vi "UserView_Entry_Console.vi"(8 "error in":errorcluster) -> (0 "error out":errorcluster)   [LabVIEW 2019]
uses:
  #typedef_Queue_enum.ctl
  #typedef_EntryConsole_Action_enum.ctl
  #typedef_Data_Controller.ctl
  #typedef_WashDisplay_Action_enum.ctl
  #typedef_Controller_Action_enum.ctl
  #typedef_VehiclePosition_Action_enum.ctl
  #typedef_VehiclePos_enum.ctl
  #typedef_WashStepInfo.ctl
  #typedef_WashStates.ctl
  #typedef_Data_Entry.ctl
panel:
  in  "Start":bool
  in  "Air Dry":bool
  in  "Tire Shine Foam":bool
  in  "Spot Free Rinse":bool
  in  "Low Pressure Wax":bool
  in  "High Pressure Wash (default)":bool
  in  "Pre-Soak":bool
  in  "Bug Remover":bool
  in  "Under Body Wash":bool
  # "Entry Console"
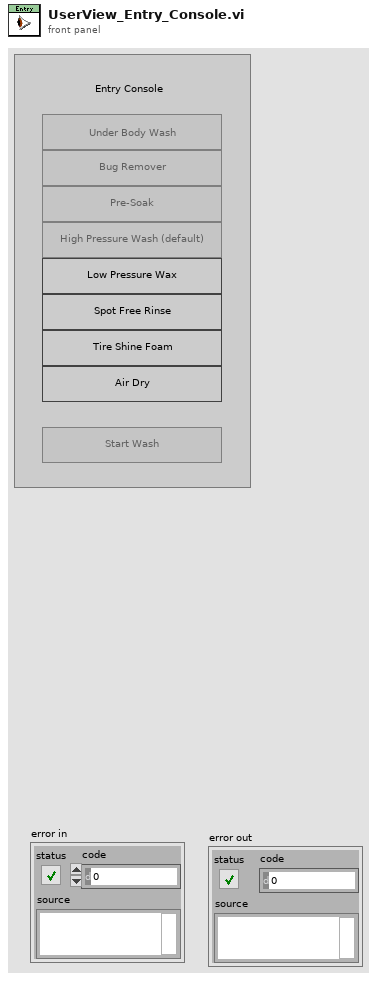
[diagram p1: front panel]
types:
  T1 = typedef "#typedef_Queue_enum.ctl" = enum16{"ERROR_default", "Obtain", "Enqueue", "GetStatus", "Flush", "Release"}
  T2 = typedef "#typedef_Data_Entry.ctl" = cluster{"Under Body Wash":bool, "Bug Remover":bool, "Pre-Soak":bool, "High Pressure Wash (default)":bool, "Low Pressure Wax":bool, "Spot Free Rinse":bool, "Tire Shine Foam":bool, "Air Dry":bool, "Start":bool, "EntryConsole_Action":T3}
  T3 = typedef "#typedef_EntryConsole_Action_enum.ctl" = enum16{"Init", "ERROR_DEFAULT", "Idle", "Start_Wash_Cycle", "Clear_Console", "Close", "Error_Handler", "Exit"}
  T4 = typedef "#typedef_Data_Controller.ctl" = cluster{"EntryConsole_Action":T3, "WashDisplay_Action":T5, "Controller_Action":T6, "VehiclePosition_Action":T7, "Under Body Wash":bool, "Bug Remover":bool, "Pre-Soak":bool, "High Pressure Wash (default)":bool, "Low Pressure Wax":bool, "Spot Free Rinse":bool, "Tire Shine Foam":bool, "Air Dry":bool, "Start":bool, "Current Vehicle Pos":T8, "Steps List":T9[], "Current Step Ind":i32}
  T5 = typedef "#typedef_WashDisplay_Action_enum.ctl" = enum16{"Init", "ERROR_DEFAULT", "Idle", "Update FP", "Close", "Error_Handler", "Exit"}
  T6 = typedef "#typedef_Controller_Action_enum.ctl" = enum16{"ERROR_DEFAULT", "Init", "Read database", "(Idle) Wait for Start", "Start", "Wait for Vehicle Pos", "Wash Step Execution", "Wash Completion", "Wash Exit", "Wash Abort", "Close", "Error Handler", "Exit"}
  T7 = typedef "#typedef_VehiclePosition_Action_enum.ctl" = enum16{"Init", "ERROR_DEFAULT", "Idle", "Close", "Error_Handler", "Exit", "Send Vehicle Pos"}
  T8 = typedef "#typedef_VehiclePos_enum.ctl" = u8
  T9 = typedef "#typedef_WashStepInfo.ctl" = cluster{"Wash States":T10, "Expected Vehicle Pos":i32, "Step duration":i32}
  T10 = typedef "#typedef_WashStates.ctl" = enum16{"Under Body Wash", "Bug Remover", "Pre-Soak", "High Pressure Wash", "Low Pressure Wax", "Spot Free Rinse", "Tire Shine Foam", "Air Dry"}
  T11 = enum8{"Enabled", "Disabled", "Disabled and Grayed Out"}
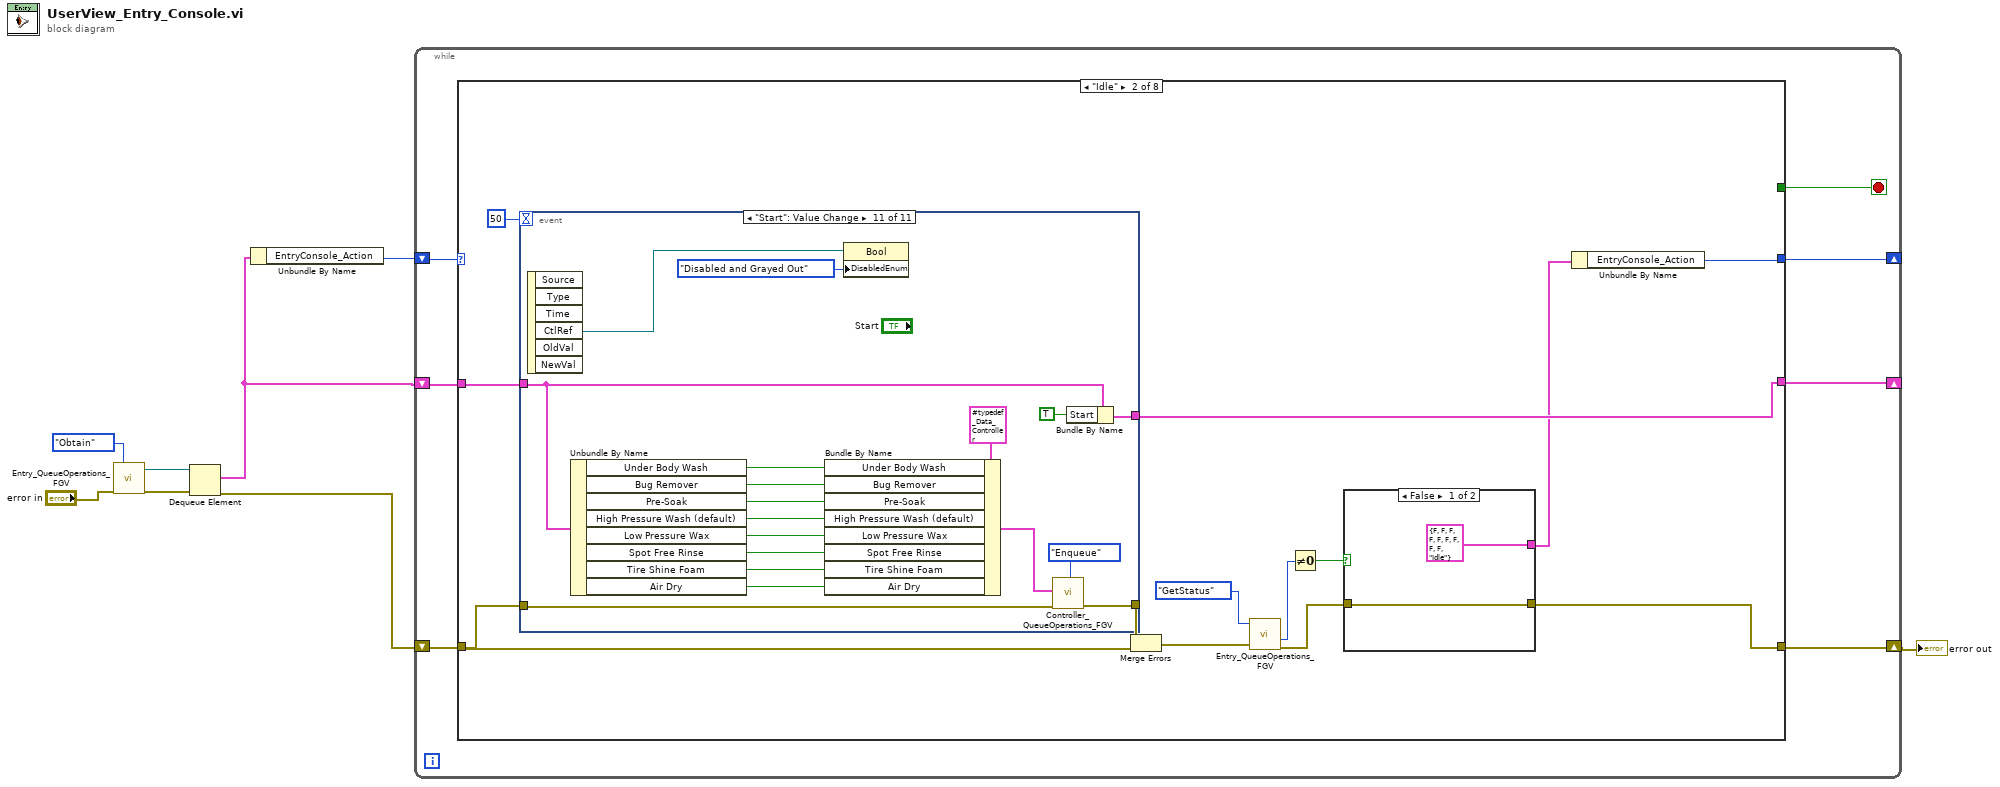
[diagram p0: block diagram]
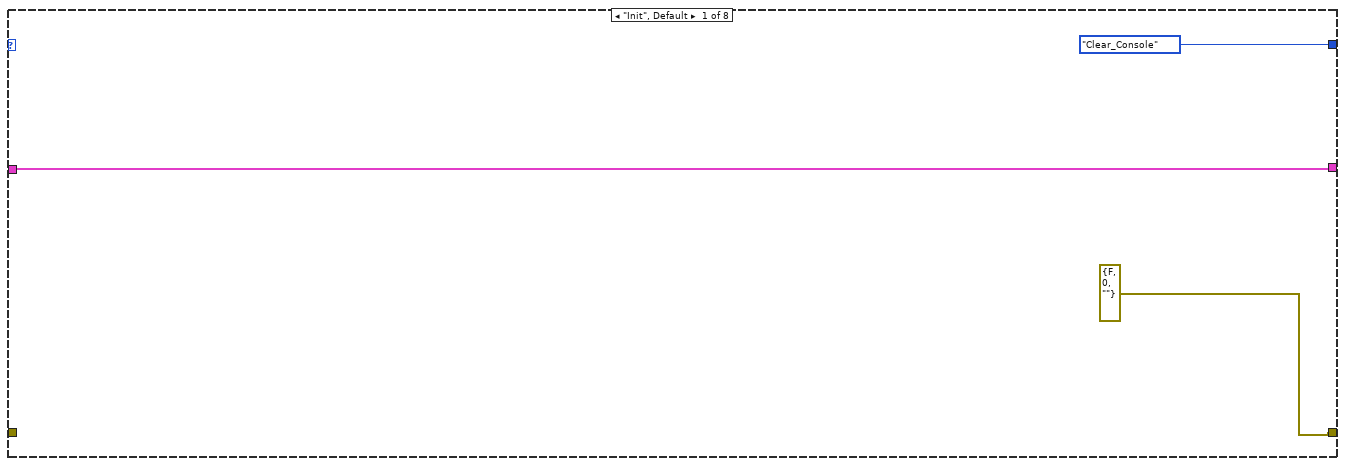
[diagram p2: hidden frame]
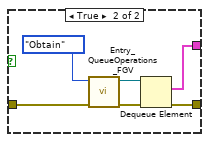
[diagram p3: hidden frame]
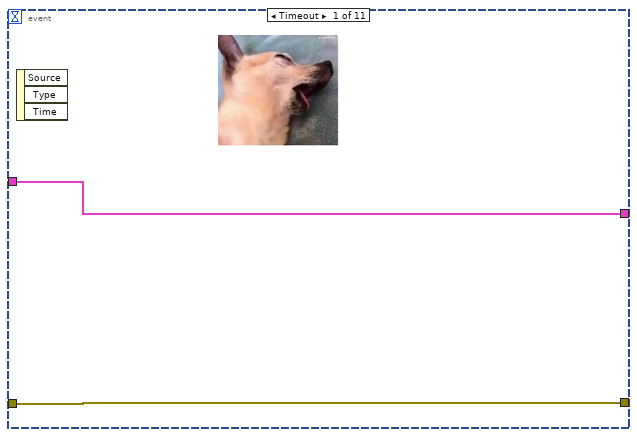
[diagram p4: hidden frame]
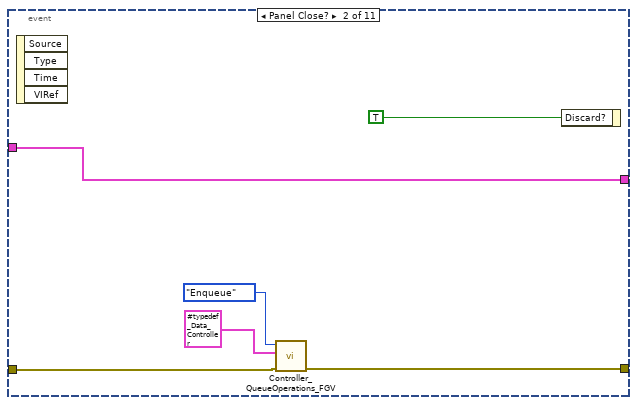
[diagram p5: hidden frame]
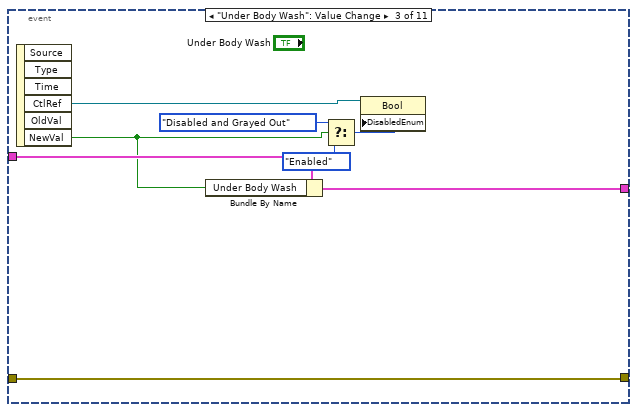
[diagram p6: hidden frame]
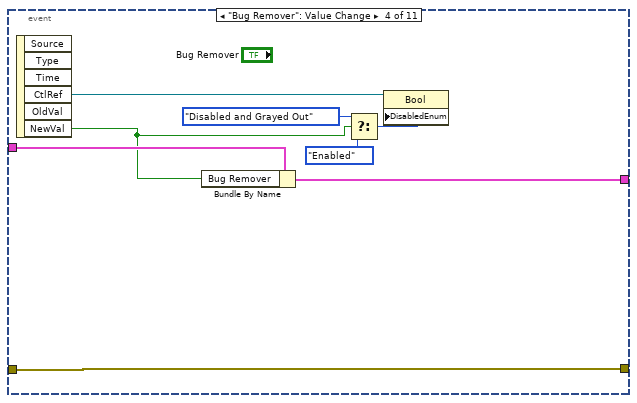
[diagram p7: hidden frame]
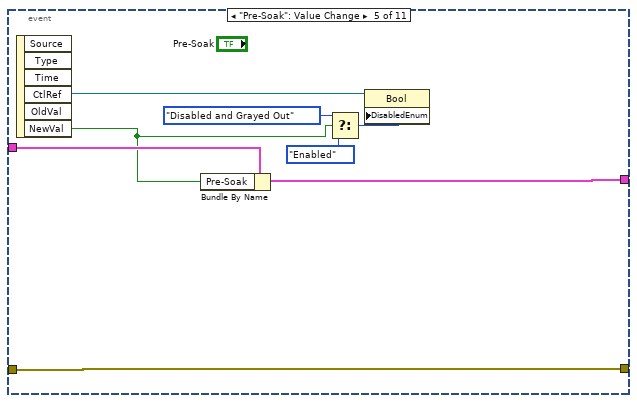
[diagram p8: hidden frame]
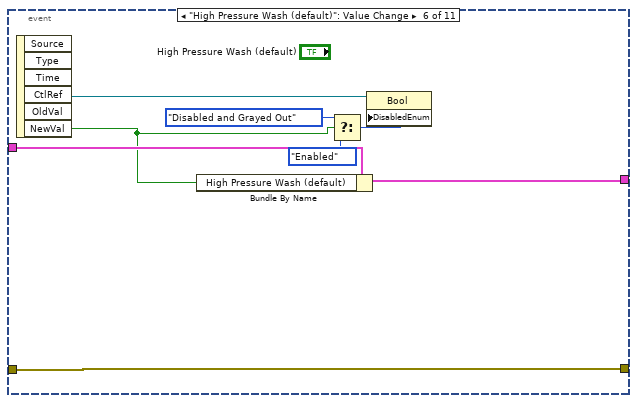
[diagram p9: hidden frame]
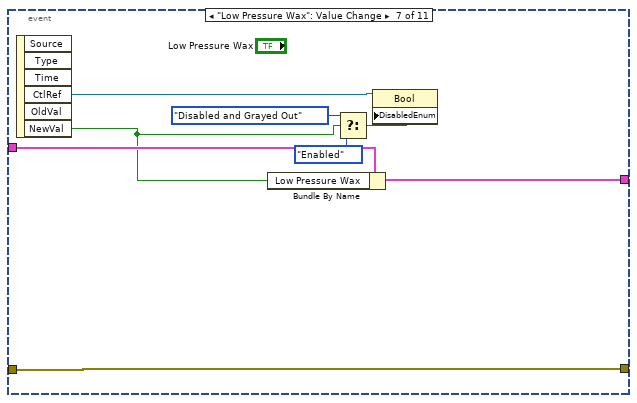
[diagram p10: hidden frame]
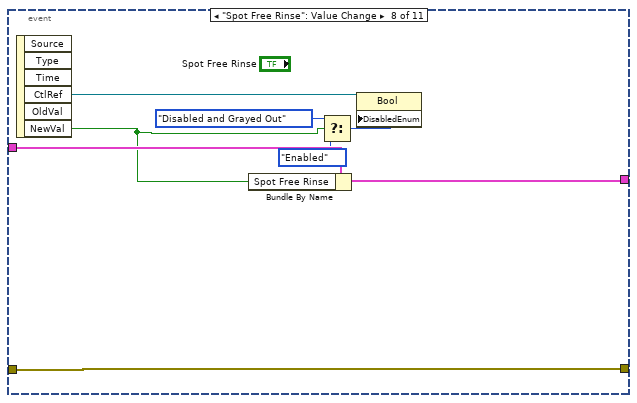
[diagram p11: hidden frame]
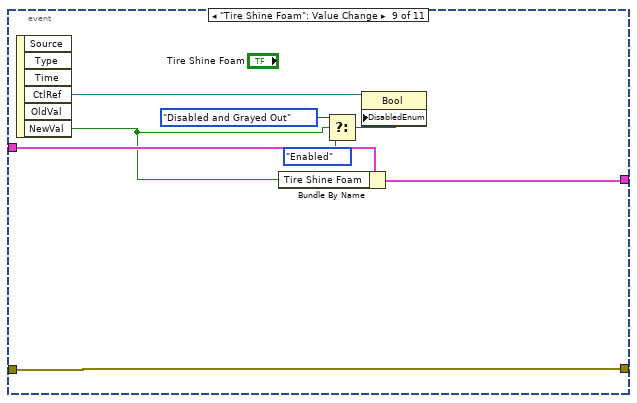
[diagram p12: hidden frame]
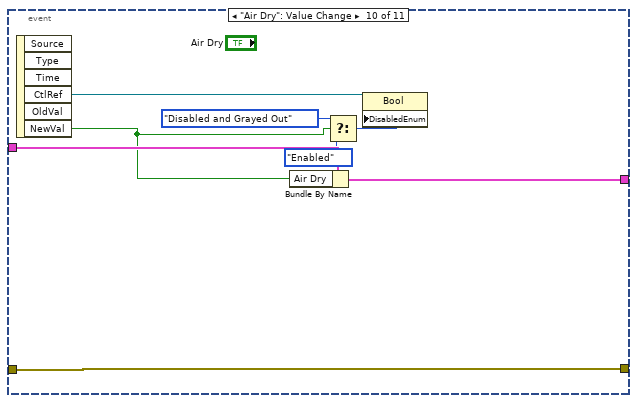
[diagram p13: hidden frame]
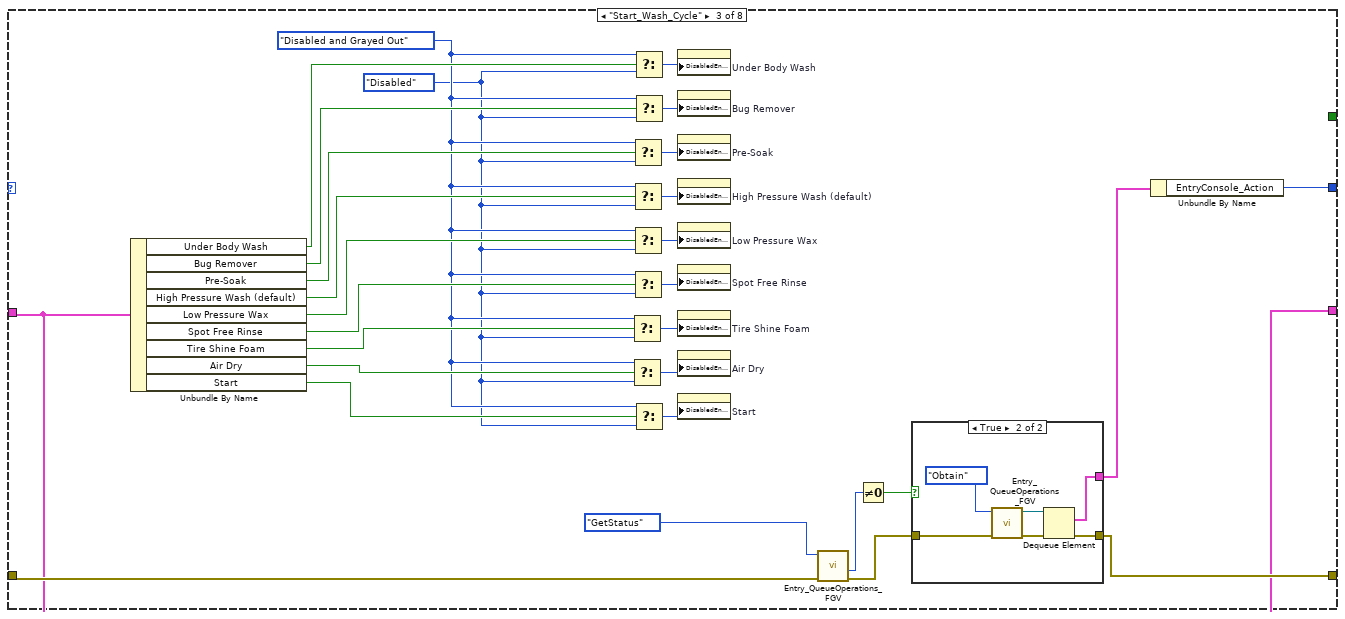
[diagram p14: hidden frame]
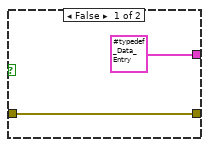
[diagram p15: hidden frame]
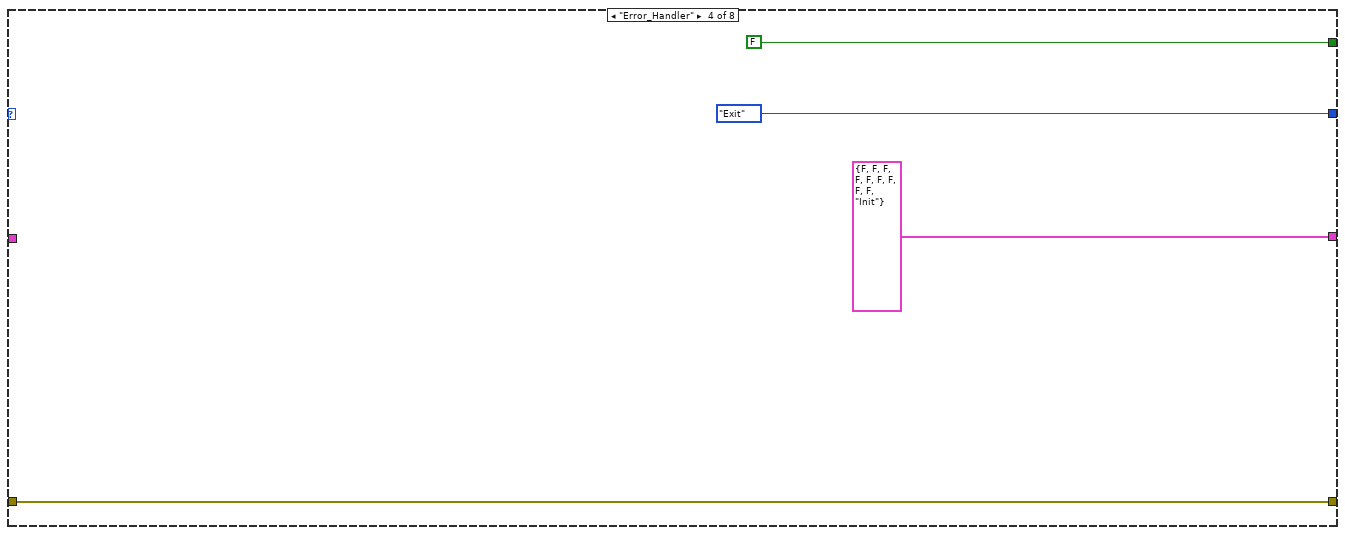
[diagram p16: hidden frame]
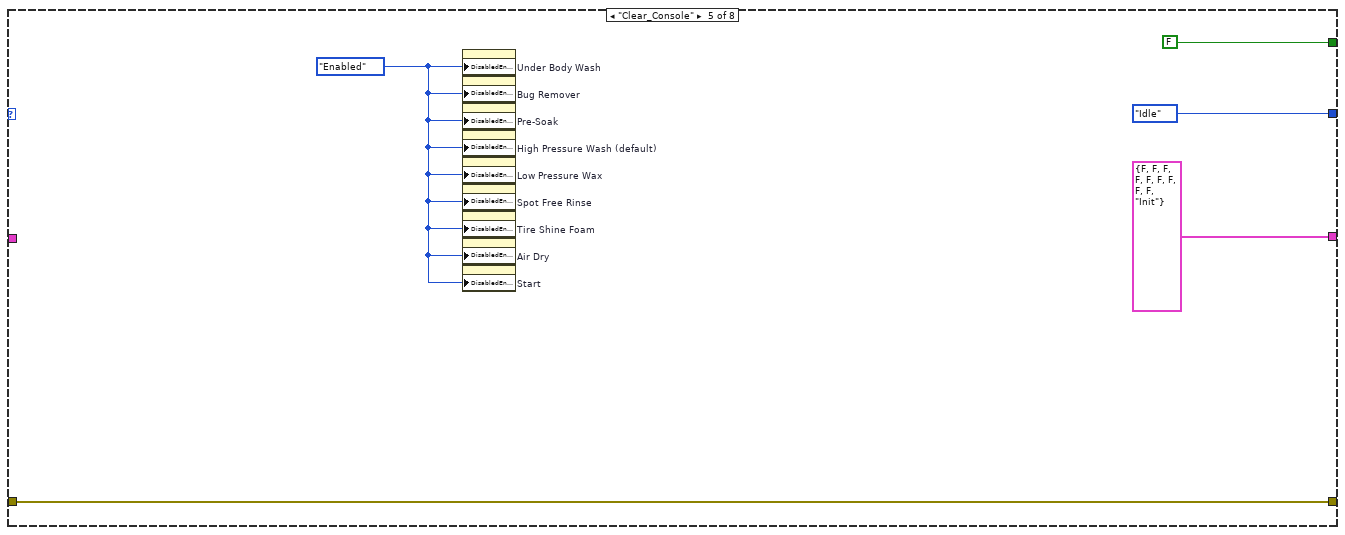
[diagram p17: hidden frame]
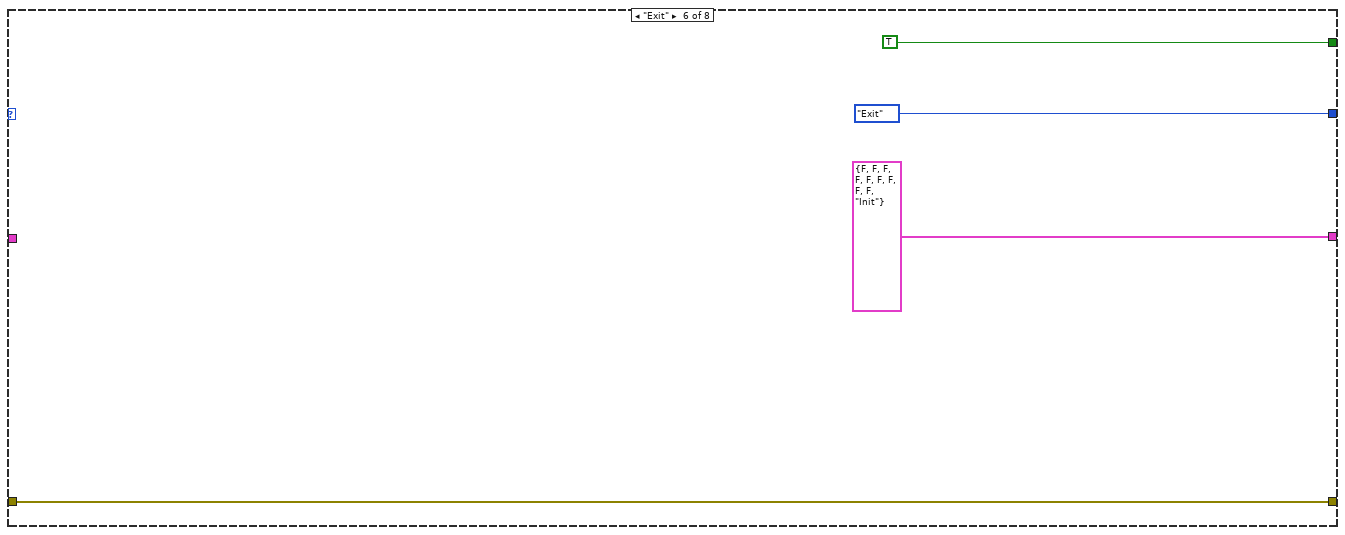
[diagram p18: hidden frame]
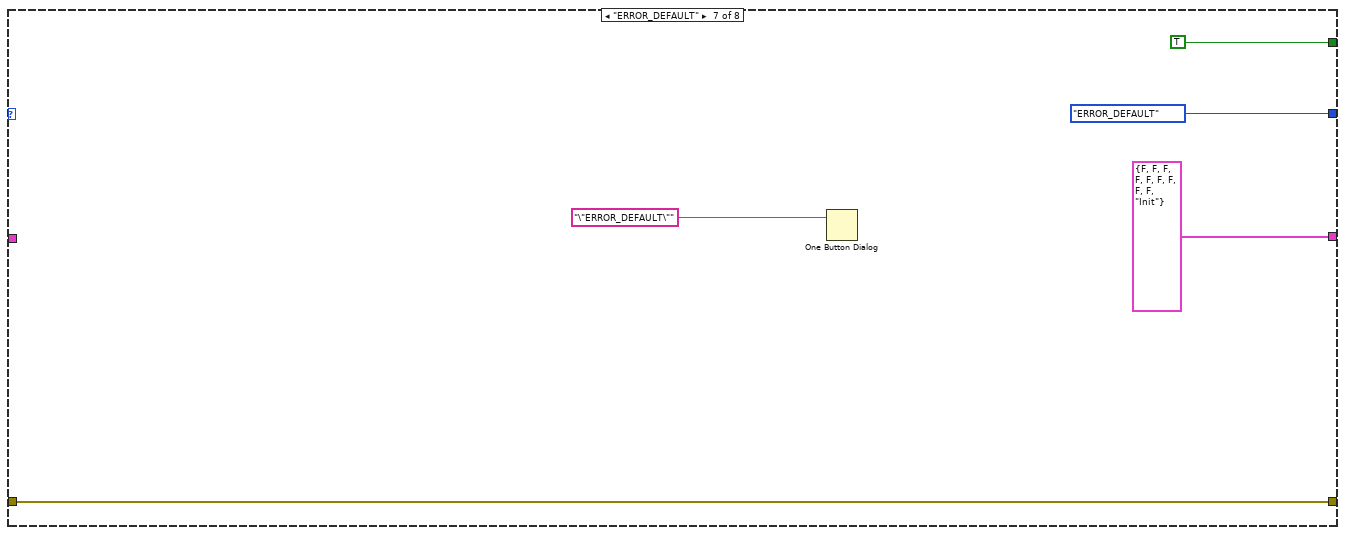
[diagram p19: hidden frame]
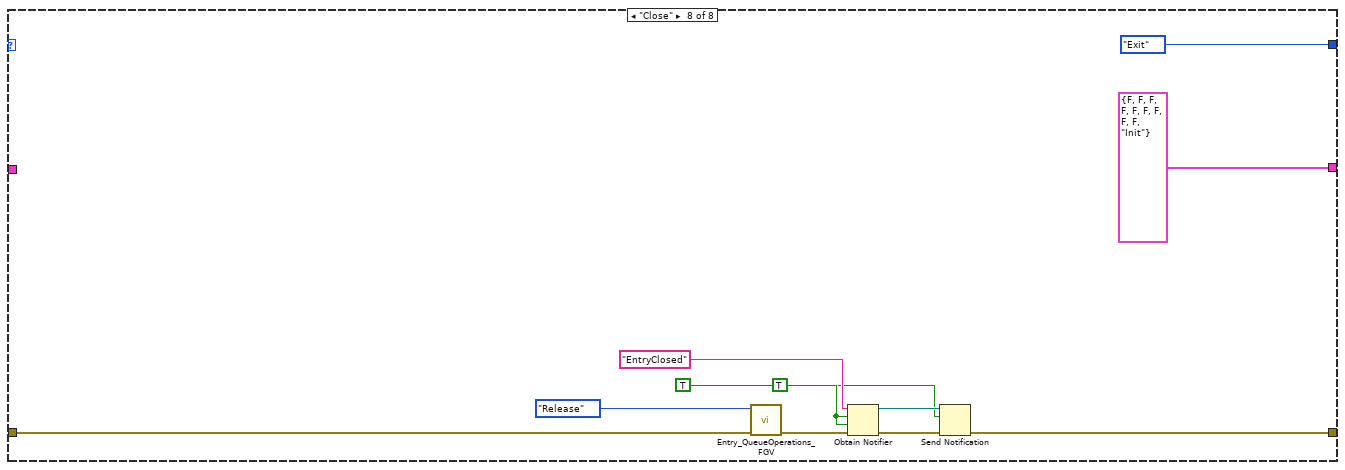
[diagram p20: hidden frame]
diagram:
  n1 = call "Entry_QueueOperations_FGV.vi"("error in"="error in", "Action"=#typedef_Queue_enum."Obtain") -> ("error out"=w5:errorcluster, "queue ref"=w6:refnum<queue>)  [unwired: 6 in, 2 out]
  n2 = Dequeue Element(queue=w6, error in (no error)=w5) -> (element=w4:T2, error out=w2:errorcluster)  [unwired: 1 in, 2 out]
  n3 = Unbundle By Name(w4) -> ("EntryConsole_Action"=w3:T3)
  n4 = while {
    shift-right: [w14] -> _
    shift-left: w3 -> [w15]
    shift-right: [w12] -> _
    shift-left: w4 -> [w9]
    shift-right: [w10] -> w1
    shift-left: w2 -> [w11]
    stop <- w13 stop-if-true
    n5 = case shown="\"Idle\"" w15 {
      tunnel: [#typedef_EntryConsole_Action_enum."Clear_Console" w25 w131 #typedef_EntryConsole_Action_enum."Exit" #typedef_EntryConsole_Action_enum."Idle" #typedef_EntryConsole_Action_enum."Exit" #typedef_EntryConsole_Action_enum."ERROR_DEFAULT" #typedef_EntryConsole_Action_enum."Exit"] -> w14
      tunnel: [_ _ _ FALSE FALSE TRUE TRUE _] -> w13
      tunnel: [w16 w26 w130 T2 {"Under Body Wash"=FALSE, "Bug Remover"=FALSE, "Pre-Soak"=FALSE, "High Pressure Wash (default)"=FALSE, "Low Pressure Wax"=FALSE, "Spot Free Rinse"=FALSE, "Tire Shine Foam"=FALSE, "Air Dry"=FALSE, "Start"=FALSE, "EntryConsole_Action"=enum."Init"} ("Data") T2 {"Under Body Wash"=FALSE, "Bug Remover"=FALSE, "Pre-Soak"=FALSE, "High Pressure Wash (default)"=FALSE, "Low Pressure Wax"=FALSE, "Spot Free Rinse"=FALSE, "Tire Shine Foam"=FALSE, "Air Dry"=FALSE, "Start"=FALSE, "EntryConsole_Action"=enum."Init"} ("Data") T2 {"Under Body Wash"=FALSE, "Bug Remover"=FALSE, "Pre-Soak"=FALSE, "High Pressure Wash (default)"=FALSE, "Low Pressure Wax"=FALSE, "Spot Free Rinse"=FALSE, "Tire Shine Foam"=FALSE, "Air Dry"=FALSE, "Start"=FALSE, "EntryConsole_Action"=enum."Init"} ("Data") T2 {"Under Body Wash"=FALSE, "Bug Remover"=FALSE, "Pre-Soak"=FALSE, "High Pressure Wash (default)"=FALSE, "Low Pressure Wax"=FALSE, "Spot Free Rinse"=FALSE, "Tire Shine Foam"=FALSE, "Air Dry"=FALSE, "Start"=FALSE, "EntryConsole_Action"=enum."Init"} ("Data") T2 {"Under Body Wash"=FALSE, "Bug Remover"=FALSE, "Pre-Soak"=FALSE, "High Pressure Wash (default)"=FALSE, "Low Pressure Wax"=FALSE, "Spot Free Rinse"=FALSE, "Tire Shine Foam"=FALSE, "Air Dry"=FALSE, "Start"=FALSE, "EntryConsole_Action"=enum."Init"} ("Data")] -> w12
      tunnel: w11 -> [_ w28 w132 w168 w173 w178 w181 w192]
      tunnel: [errorcluster {"status"=FALSE, "code"=0, "source"=""} ("error constant") w21 w133 w168 w173 w178 w181 w188] -> w10
      tunnel: w9 -> [w16 w27 w130 _ _ _ _ _]
      frame "Init", Default {
      }
      frame "Idle" {
        n6 = event shown="[10] \"Start\": Value Change" {
          selector: _ -> [_ _ _ _ _ _ _ _ _ _ _]
          dyn-events: _ -> [_ _ _ _ _ _ _ _ _ _ _]
          timeout: 50 -> [_ _ _ _ _ _ _ _ _ _ _]
          tunnel: w28 -> [w41 w45 w55 w63 w71 w79 w87 w95 w103 w111 w112]
          tunnel: [w41 w44 w55 w63 w71 w79 w87 w95 w103 w111 w125] -> w29
          tunnel: w27 -> [w40 w42 w54 w62 w70 w78 w86 w94 w102 w110 w122]
          tunnel: [w40 w42 w53 w61 w69 w77 w85 w93 w101 w109 w123] -> w26
          event Timeout {
            n7 = event-data() -> ()  [unwired: 1 in, 3 out]
          }
          event Panel Close? {
            n8 = event-data() -> ()  [unwired: 1 in, 4 out]
            n9 = call "Controller_QueueOperations_FGV.vi"("error in"=w45, "Data In"=T4 {"EntryConsole_Action"=enum."Init", "WashDisplay_Action"=enum."Init", "Controller_Action"=enum."Close", "VehiclePosition_Action"=enum."Init", "Under Body Wash"=FALSE, "Bug Remover"=FALSE, "Pre-Soak"=FALSE, "High Pressure Wash (default)"=FALSE, "Low Pressure Wax"=FALSE, "Spot Free Rinse"=FALSE, "Tire Shine Foam"=FALSE, "Air Dry"=FALSE, "Start"=FALSE, "Current Vehicle Pos"=1, "Steps List"=[], "Current Step Ind"=0} ("Data"), "Action"=#typedef_Queue_enum."Enqueue") -> ("error out"=w44:errorcluster)  [unwired: 5 in, 3 out]
            n10 = event-data("Discard?"=TRUE) -> ()  [unwired: 1 in, 1 out]
          }
          event "Under Body Wash": Value Change {
            n11 = event-data() -> ("CtlRef"=w49:refnum<vi>, "NewVal"=w48:bool)  [unwired: 1 in, 4 out]
            n12 = Bundle By Name(cluster=w54, "Under Body Wash"=w48) -> (w53:T2)
            n13 = Select(t=T11."Disabled and Grayed Out" ("Disabled"), s=w48, f=T11."Enabled") -> (s? t:f=w51:T11)
            n14 = property class="Bool"(reference=w49, "DisabledEnum"=w51) -> ()  [unwired: 1 in, 2 out]
          }
          event "Bug Remover": Value Change {
            n15 = event-data() -> ("CtlRef"=w60:refnum<vi>, "NewVal"=w56:bool)  [unwired: 1 in, 4 out]
            n16 = Bundle By Name(cluster=w62, "Bug Remover"=w56) -> (w61:T2)
            n17 = Select(t=T11."Disabled and Grayed Out" ("Disabled"), s=w56, f=T11."Enabled") -> (s? t:f=w58:T11)
            n18 = property class="Bool"(reference=w60, "DisabledEnum"=w58) -> ()  [unwired: 1 in, 2 out]
          }
          event "Pre-Soak": Value Change {
            n19 = event-data() -> ("CtlRef"=w65:refnum<vi>, "NewVal"=w64:bool)  [unwired: 1 in, 4 out]
            n20 = Bundle By Name(cluster=w70, "Pre-Soak"=w64) -> (w69:T2)
            n21 = Select(t=T11."Disabled and Grayed Out" ("Disabled"), s=w64, f=T11."Enabled") -> (s? t:f=w67:T11)
            n22 = property class="Bool"(reference=w65, "DisabledEnum"=w67) -> ()  [unwired: 1 in, 2 out]
          }
          event "High Pressure Wash (default)": Value Change {
            n23 = event-data() -> ("CtlRef"=w73:refnum<vi>, "NewVal"=w72:bool)  [unwired: 1 in, 4 out]
            n24 = Bundle By Name(cluster=w78, "High Pressure Wash (default)"=w72) -> (w77:T2)
            n25 = Select(t=T11."Disabled and Grayed Out" ("Disabled"), s=w72, f=T11."Enabled") -> (s? t:f=w75:T11)
            n26 = property class="Bool"(reference=w73, "DisabledEnum"=w75) -> ()  [unwired: 1 in, 2 out]
          }
          event "Low Pressure Wax": Value Change {
            n27 = event-data() -> ("CtlRef"=w81:refnum<vi>, "NewVal"=w80:bool)  [unwired: 1 in, 4 out]
            n28 = Bundle By Name(cluster=w86, "Low Pressure Wax"=w80) -> (w85:T2)
            n29 = Select(t=T11."Disabled and Grayed Out" ("Disabled"), s=w80, f=T11."Enabled") -> (s? t:f=w83:T11)
            n30 = property class="Bool"(reference=w81, "DisabledEnum"=w83) -> ()  [unwired: 1 in, 2 out]
          }
          event "Spot Free Rinse": Value Change {
            n31 = event-data() -> ("CtlRef"=w89:refnum<vi>, "NewVal"=w88:bool)  [unwired: 1 in, 4 out]
            n32 = Bundle By Name(cluster=w94, "Spot Free Rinse"=w88) -> (w93:T2)
            n33 = Select(t=T11."Disabled and Grayed Out" ("Disabled"), s=w88, f=T11."Enabled") -> (s? t:f=w91:T11)
            n34 = property class="Bool"(reference=w89, "DisabledEnum"=w91) -> ()  [unwired: 1 in, 2 out]
          }
          event "Tire Shine Foam": Value Change {
            n35 = event-data() -> ("CtlRef"=w97:refnum<vi>, "NewVal"=w96:bool)  [unwired: 1 in, 4 out]
            n36 = Bundle By Name(cluster=w102, "Tire Shine Foam"=w96) -> (w101:T2)
            n37 = Select(t=T11."Disabled and Grayed Out" ("Disabled"), s=w96, f=T11."Enabled") -> (s? t:f=w99:T11)
            n38 = property class="Bool"(reference=w97, "DisabledEnum"=w99) -> ()  [unwired: 1 in, 2 out]
          }
          event "Air Dry": Value Change {
            n39 = event-data() -> ("CtlRef"=w105:refnum<vi>, "NewVal"=w104:bool)  [unwired: 1 in, 4 out]
            n40 = Bundle By Name(cluster=w110, "Air Dry"=w104) -> (w109:T2)
            n41 = Select(t=T11."Disabled and Grayed Out" ("Disabled"), s=w104, f=T11."Enabled") -> (s? t:f=w107:T11)
            n42 = property class="Bool"(reference=w105, "DisabledEnum"=w107) -> ()  [unwired: 1 in, 2 out]
          }
          event "Start": Value Change {
            n43 = event-data() -> ("CtlRef"=w127:refnum<vi>)  [unwired: 1 in, 5 out]
            n44 = Unbundle By Name(w122) -> ("Under Body Wash"=w120:bool, "Bug Remover"=w119:bool, "Pre-Soak"=w118:bool, "High Pressure Wash (default)"=w117:bool, "Low Pressure Wax"=w116:bool, "Spot Free Rinse"=w115:bool, "Tire Shine Foam"=w114:bool, "Air Dry"=w113:bool)
            n45 = Bundle By Name(cluster=T4 {"EntryConsole_Action"=enum."Init", "WashDisplay_Action"=enum."Init", "Controller_Action"=enum."Start", "VehiclePosition_Action"=enum."Init", "Under Body Wash"=FALSE, "Bug Remover"=FALSE, "Pre-Soak"=FALSE, "High Pressure Wash (default)"=FALSE, "Low Pressure Wax"=FALSE, "Spot Free Rinse"=FALSE, "Tire Shine Foam"=FALSE, "Air Dry"=FALSE, "Start"=FALSE, "Current Vehicle Pos"=1, "Steps List"=[], "Current Step Ind"=0} ("Data"), "Under Body Wash"=w120, "Bug Remover"=w119, "Pre-Soak"=w118, "High Pressure Wash (default)"=w117, "Low Pressure Wax"=w116, "Spot Free Rinse"=w115, "Tire Shine Foam"=w114, "Air Dry"=w113) -> (w121:T4)
            n46 = property class="Bool"(reference=w127, "DisabledEnum"=T11."Disabled and Grayed Out" ("Disabled")) -> ()  [unwired: 1 in, 2 out]
            n47 = call "Controller_QueueOperations_FGV.vi"("error in"=w112, "Data In"=w121, "Action"=#typedef_Queue_enum."Enqueue") -> ("error out"=w125:errorcluster)  [unwired: 5 in, 3 out]
            n48 = Bundle By Name(cluster=w122, "Start"=TRUE ("Under Body Wash")) -> (w123:T2)
          }
        }
        n49 = Merge Errors(w29, w28) -> (w30:errorcluster)
        n50 = call "Entry_QueueOperations_FGV.vi"("error in"=w30, "Action"=#typedef_Queue_enum."GetStatus") -> ("error out"=w22:errorcluster, "#elements in queue"=w23:i32)  [unwired: 6 in, 2 out]
        n51 = Not Equal To 0?(x=w23) -> (x != 0?=w24:bool)
        n52 = case shown="False" w24 {
          tunnel: w22 -> [w33 w38]
          tunnel: [w33 w36] -> w21
          tunnel: [T2 {"Under Body Wash"=FALSE, "Bug Remover"=FALSE, "Pre-Soak"=FALSE, "High Pressure Wash (default)"=FALSE, "Low Pressure Wax"=FALSE, "Spot Free Rinse"=FALSE, "Tire Shine Foam"=FALSE, "Air Dry"=FALSE, "Start"=FALSE, "EntryConsole_Action"=enum."Idle"} ("Data") w34] -> w20
          frame False {
          }
          frame True {
            n53 = call "Entry_QueueOperations_FGV.vi"("error in"=w38, "Action"=#typedef_Queue_enum."Obtain") -> ("error out"=w37:errorcluster, "queue ref"=w35:refnum<queue>)  [unwired: 6 in, 2 out]
            n54 = Dequeue Element(queue=w35, error in (no error)=w37) -> (element=w34:T2, error out=w36:errorcluster)  [unwired: 1 in, 2 out]
          }
        }
        n55 = Unbundle By Name(w20) -> ("EntryConsole_Action"=w25:T3)
      }
      frame "Start_Wash_Cycle" {
        w148 = T11."Disabled" ("f")
        w149 = T11."Disabled and Grayed Out" ("Disabled")
        n56 = Unbundle By Name(w130) -> ("Under Body Wash"=w158:bool, "Bug Remover"=w157:bool, "Pre-Soak"=w156:bool, "High Pressure Wash (default)"=w155:bool, "Low Pressure Wax"=w154:bool, "Spot Free Rinse"=w153:bool, "Tire Shine Foam"=w152:bool, "Air Dry"=w151:bool, "Start"=w150:bool)
        n57 = Select(t=w149, s=w152, f=w148) -> (s? t:f=w141:T11)
        n58 = Select(t=w149, s=w151, f=w148) -> (s? t:f=w140:T11)
        n59 = Select(t=w149, s=w156, f=w148) -> (s? t:f=w145:T11)
        n60 = Select(t=w149, s=w155, f=w148) -> (s? t:f=w144:T11)
        n61 = Select(t=w149, s=w154, f=w148) -> (s? t:f=w143:T11)
        n62 = Select(t=w149, s=w153, f=w148) -> (s? t:f=w142:T11)
        n63 = Select(t=w149, s=w158, f=w148) -> (s? t:f=w147:T11)
        n64 = Select(t=w149, s=w157, f=w148) -> (s? t:f=w146:T11)
        n65 = Select(t=w149, s=w150, f=w148) -> (s? t:f=w139:T11)
        n66 = property on="Under Body Wash" class="Bool"("DisabledEnum"=w147) -> ()  [unwired: 2 in, 2 out]
        n67 = property on="Bug Remover" class="Bool"("DisabledEnum"=w146) -> ()  [unwired: 2 in, 2 out]
        n68 = property on="Pre-Soak" class="Bool"("DisabledEnum"=w145) -> ()  [unwired: 2 in, 2 out]
        n69 = property on="High Pressure Wash (default)" class="Bool"("DisabledEnum"=w144) -> ()  [unwired: 2 in, 2 out]
        n70 = property on="Low Pressure Wax" class="Bool"("DisabledEnum"=w143) -> ()  [unwired: 2 in, 2 out]
        n71 = property on="Spot Free Rinse" class="Bool"("DisabledEnum"=w142) -> ()  [unwired: 2 in, 2 out]
        n72 = property on="Tire Shine Foam" class="Bool"("DisabledEnum"=w141) -> ()  [unwired: 2 in, 2 out]
        n73 = property on="Air Dry" class="Bool"("DisabledEnum"=w140) -> ()  [unwired: 2 in, 2 out]
        n74 = property on="Start" class="Bool"("DisabledEnum"=w139) -> ()  [unwired: 2 in, 2 out]
        n75 = call "Entry_QueueOperations_FGV.vi"("error in"=w132, "Action"=#typedef_Queue_enum."GetStatus") -> ("error out"=w135:errorcluster, "#elements in queue"=w136:i32)  [unwired: 6 in, 2 out]
        n76 = Not Equal To 0?(x=w136) -> (x != 0?=w137:bool)
        n77 = case shown="True" w137 {
          tunnel: w135 -> [w160 w165]
          tunnel: [w160 w163] -> w133
          tunnel: [T2 {"Under Body Wash"=FALSE, "Bug Remover"=FALSE, "Pre-Soak"=FALSE, "High Pressure Wash (default)"=FALSE, "Low Pressure Wax"=FALSE, "Spot Free Rinse"=FALSE, "Tire Shine Foam"=FALSE, "Air Dry"=FALSE, "Start"=FALSE, "EntryConsole_Action"=enum."Start_Wash_Cycle"} ("Data") w161] -> w134
          frame False {
          }
          frame True {
            n78 = call "Entry_QueueOperations_FGV.vi"("error in"=w165, "Action"=#typedef_Queue_enum."Obtain") -> ("error out"=w164:errorcluster, "queue ref"=w162:refnum<queue>)  [unwired: 6 in, 2 out]
            n79 = Dequeue Element(queue=w162, error in (no error)=w164) -> (element=w161:T2, error out=w163:errorcluster)  [unwired: 1 in, 2 out]
          }
        }
        n80 = Unbundle By Name(w134) -> ("EntryConsole_Action"=w131:T3)
      }
      frame "Error_Handler" {
      }
      frame "Clear_Console" {
        w171 = T11."Enabled" ("Disabled")
        n81 = property on="Under Body Wash" class="Bool"("DisabledEnum"=w171) -> ()  [unwired: 2 in, 2 out]
        n82 = property on="Bug Remover" class="Bool"("DisabledEnum"=w171) -> ()  [unwired: 2 in, 2 out]
        n83 = property on="Pre-Soak" class="Bool"("DisabledEnum"=w171) -> ()  [unwired: 2 in, 2 out]
        n84 = property on="High Pressure Wash (default)" class="Bool"("DisabledEnum"=w171) -> ()  [unwired: 2 in, 2 out]
        n85 = property on="Low Pressure Wax" class="Bool"("DisabledEnum"=w171) -> ()  [unwired: 2 in, 2 out]
        n86 = property on="Spot Free Rinse" class="Bool"("DisabledEnum"=w171) -> ()  [unwired: 2 in, 2 out]
        n87 = property on="Tire Shine Foam" class="Bool"("DisabledEnum"=w171) -> ()  [unwired: 2 in, 2 out]
        n88 = property on="Air Dry" class="Bool"("DisabledEnum"=w171) -> ()  [unwired: 2 in, 2 out]
        n89 = property on="Start" class="Bool"("DisabledEnum"=w171) -> ()  [unwired: 2 in, 2 out]
      }
      frame "Exit" {
      }
      frame "ERROR_DEFAULT" {
        n90 = One Button Dialog(message="\"ERROR_DEFAULT\"") -> ()  [unwired: 1 in, 1 out]
      }
      frame "Close" {
        w189 = TRUE
        n91 = call "Entry_QueueOperations_FGV.vi"("error in"=w192, "Action"=#typedef_Queue_enum."Release") -> ("error out"=w193:errorcluster)  [unwired: 6 in, 3 out]
        n92 = Obtain Notifier(name (unnamed)="EntryClosed", notification data type=w189, create if not found? (T)=w189, error in (no error)=w193) -> (notifier out=w187:refnum<notifier>, error out=w191:errorcluster)  [unwired: 1 out]
        n93 = Send Notification(notification=TRUE, notifier=w187, error in (no error)=w191) -> (error out=w188:errorcluster)  [unwired: 1 out]
      }
    }
  }
  "error out" <- w1
